vi "Client.vi"() -> ()   [LabVIEW 2021]
doc: "This VI acts as a client for an incoming websockets connection. Receives/sends string data to the connected client."
uses:
  StatusCode.ctl
  LV WebSockets.lvlib
panel:
  out "Status Code":T1=1000 items=["Normal Closure"=1000, "Going Away"=1001, "Protocol Error"=1002, "Wrong Data Type"=1003, "Reserved 1004"=1004, "Reserved 1005"=1005, "Reserved 1006"=1006, "Non Consistent Data Type"=1007, "Policy Violation"=1008, "Message Too Big"=1009, "Extensions Negotiation Error"=1010, "Unexpected Condition"=1011, "Reserved 1015"=1015]
  out "Close Reason":string
  in  "WS URI":string="ws://localhost:6123/resource/name"
  out "Resource Name":string
  out "HTTP Headers":variant
  in  "Stop":bool
  out "Received Data":string
  in  "Send":bool
  in  "Data":string
  # "WebSockets Example Client"
  # "This VI is a simple example of sending/receiving data using WebSockets.\nIt opens a WebSockets connection on Port 6123 and\nthen displays incoming string data. Strings can also be sent back to the client.\n\nInstructions for use:\n1) Run the SingleConnection.vi VI\n2) Set a suitable websocket URI including a resource name matching the one defined on the server\n2) Quickly run this VI"
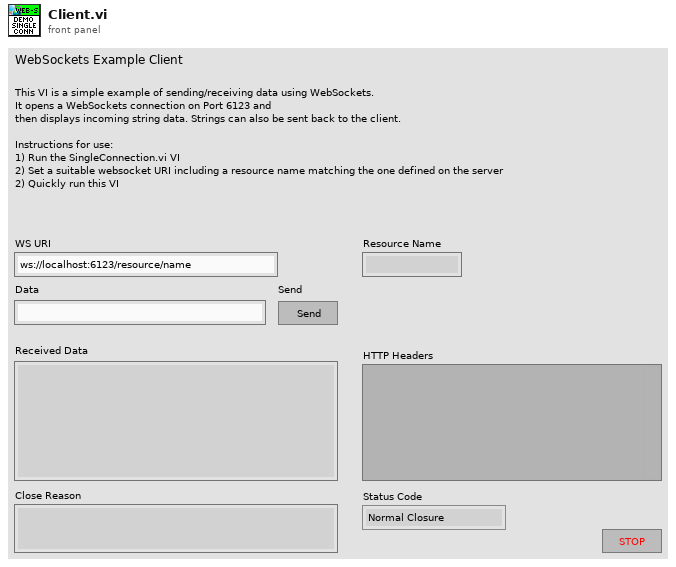
[diagram p1: front panel]
types:
  T1 = typedef "LV WebSockets.lvlib/StatusCode.ctl" = u16
  T2 = typedef "LV WebSockets.lvlib/Opcode.ctl" = enum8{"Continuation Frame", "Text Frame", "Binary Frame", "Reserved 3", "Reserved 4", "Reserved 5", "Reserved 6", "Reserved 7", "Connection Close", "Ping", "Pong", "Reserved B", "Reserved C", "Reserved D", "Reserved F"}
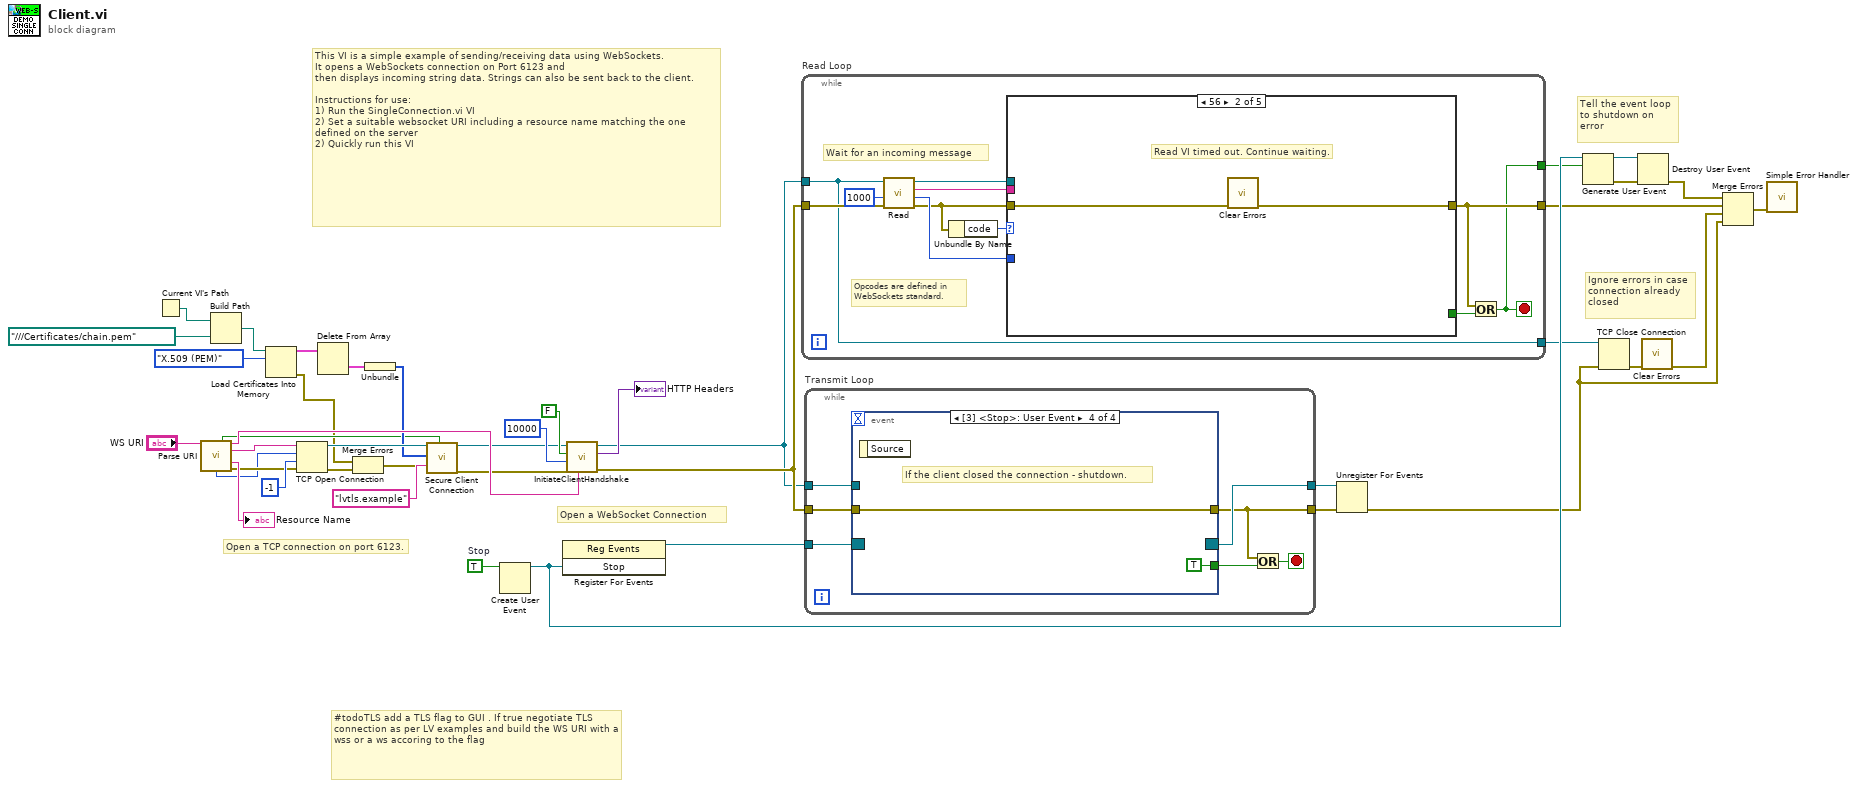
[diagram p0: block diagram]
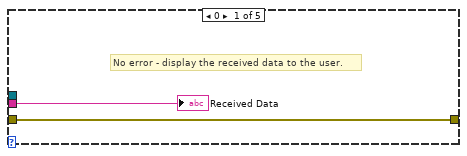
[diagram p2: hidden frame]
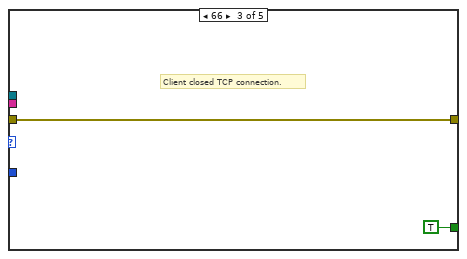
[diagram p3: hidden frame]
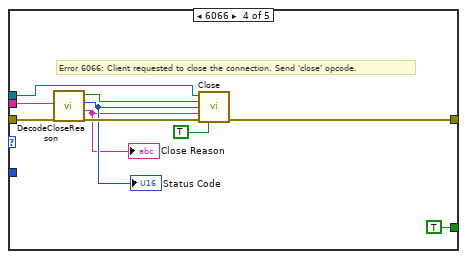
[diagram p4: hidden frame]
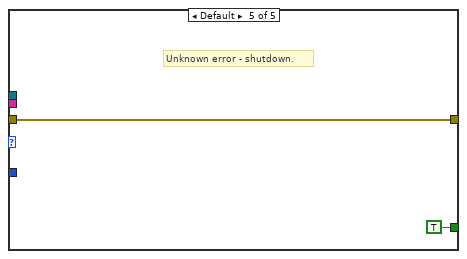
[diagram p5: hidden frame]
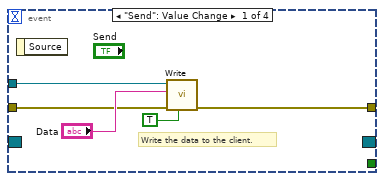
[diagram p6: hidden frame]
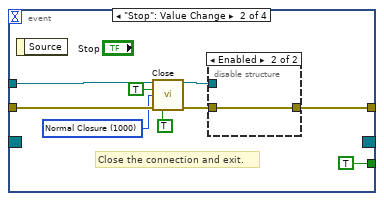
[diagram p7: hidden frame]
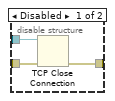
[diagram p8: hidden frame]
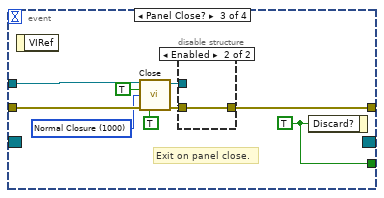
[diagram p9: hidden frame]
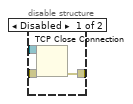
[diagram p10: hidden frame]
diagram:
  w40 = TRUE  # Stop
  # "#todoTLS add a TLS flag to GUI . If true negotiate TLS connection as per LV examples and build the WS URI with a wss or a ws accoring to the flag"
  # "Ignore errors in case\nconnection already\nclosed"
  # "Tell the event loop to shutdown on error"
  # "This VI is a simple example of sending/receiving data using WebSockets.\nIt opens a WebSockets connection on Port 6123 and\nthen displays incoming string data. Strings can also be sent back to the client.\n\nInstructions for use:\n1) Run the SingleConnection.vi VI\n2) Set a suitable websocket URI including a resource name matching the one defined on the server\n2) Quickly run this VI"
  # "Open a WebSocket Connection"
  # "Open a TCP connection on port 6123."
  n1 = Current VI's Path() -> (path=w3:path)
  n2 = call "Parse URI.vi"("URI"="WS URI") -> ("Secure"=w4:bool, "URI Out"=w24:string, "Hostname"=w23:string, "Resource Name"=→"Resource Name":string, "Port"=w19:u16, "error out"=w21:errorcluster)  [unwired: 7 in, 2 out]
  n3 = Build Path(base path=w3, name or relative path=path "../../../Certificates/chain.pem" ("cert chain")) -> (appended path=w13:path)
  n4 = Load Certificates Into Memory(10:enum32{"X.509 (PEM)"}."X.509 (PEM)" ("format"), 11:w13) -> (0:w1:errorcluster, 3:w6:cluster{"certificate":u8[]}[])  [unwired: 1 in]
  n5 = TCP Open Connection(address=w23, remote port or service name=w19, timeout ms (60000)=-1 ("timeout ms (25000)"), error in (no error)=w21) -> (connection ID=w9:refnum<k5>, error out=w12:errorcluster)  [unwired: 1 in]
  n6 = Delete From Array(array=w6) -> (deleted portion=w7:cluster{"certificate":u8[]})  [unwired: 2 in, 1 out]
  n7 = Merge Errors(w1, w12) -> (w2:errorcluster)
  n8 = Unbundle(w7) -> ("certificate"=w5:u8[])
  n9 = call "Secure Client Connection.vi"("TCP connection"=w9, "certificate"=w5, "server hostname"="lvtls.example" ("expected server hostname (must be \"lvtls.example\")"), "error in"=w2, "Secure the Connection (T)"=w4) -> ("TCP connection out"=w10:refnum<k5>, "error out"=w11:errorcluster)  [unwired: 12 in, 1 out]
  n10 = Create User Event(user event datatype=w40) -> (user event=w38:refnum<user-event>)  [unwired: 1 in, 1 out]
  n11 = register-events(w38) -> (reference out=w41:refnum<event-registration>)  [unwired: 2 in, 1 out]
  n12 = call "InitiateClientHandshake.vi"("WS URI"=w24, "error in (no error)"=w11, "timeout ms (5000)"=10000 ("timeout ms (25000)"), "Relative URI Request (F)"=FALSE, "WebSocket Connection in"=w10) -> ("error out"=w29:errorcluster, "Return Headers Out"=→"HTTP Headers":variant, "WebSocket Connection out"=w27:refnum<k5>)  [unwired: 4 in]
  n13 = while "Read Loop" {
    tunnel: w27 -> [w43]
    tunnel: [w44] -> w37
    tunnel: [w46] -> w28
    tunnel: w29 -> [w47]
    tunnel: [w43] -> w16
    stop <- w44 stop-if-true
    # "Wait for an incoming message"
    # "Opcodes are defined in\nWebSockets standard."
    n14 = call "Read.vi"("error in (no error)"=w47, "timeout ms (5000)"=1000 ("timeout ms (25000)"), "WebSocket Connection in"=w43) -> ("error out"=w48:errorcluster, "Opcode out"=w49:T2, "Data"=w51:string, "WebSocket Connection out"=w50:refnum<k5>)  [unwired: 5 in]
    n15 = Unbundle By Name(w48) -> ("code"=w52:i32)
    n16 = case shown="56" w52 {
      tunnel: w51 -> [w55 _ _ w64 _]
      tunnel: [_ _ TRUE TRUE TRUE] -> w45
      tunnel: w50 -> [_ _ _ w68 _]
      tunnel: w49 -> [_ _ _ _ _]
      tunnel: w48 -> [w54 w57 w58 w66 w69]
      tunnel: [w54 w56 w58 w65 w69] -> w46
      frame 0 {
        # "No error - display the received data to the user."
        "Received Data" <- w55
      }
      frame 56 {
        # "Read VI timed out. Continue waiting."
        n17 = call <vilib>:"Clear Errors.vi"("error in (no error)"=w57) -> ("error out"=w56:errorcluster)  [unwired: 5 in, 1 out]
      }
      frame 66 {
        # "Client closed TCP connection."
      }
      frame 6066 {
        # "Error 6066: Client requested to close the connection. Send 'close' opcode."
        n18 = call "DecodeCloseReason.vi"("Data"=w64) -> ("Reason"=w60:string, "Status Code"=w62:T1, "Close Reason Given"=w63:bool)  [unwired: 8 in]
        "Close Reason" <- w60
        "Status Code" <- w62
        n19 = call "Close.vi"("WebSocket Connection in"=w68, "Send Reason (F)"=w63, "Status Code"=w62, "Reason"=w60, "error in (no error)"=w66, "Mask payload?"=TRUE) -> ("error out"=w65:errorcluster)  [unwired: 8 in, 1 out]
      }
      frame Default {
        # "Unknown error - shutdown."
      }
    }
    n20 = Or(x=w46, y=w45) -> (x .or. y?=w44:bool)
  }
  n21 = while "Transmit Loop" {
    tunnel: w27 -> [w77]
    tunnel: w41 -> [w76]
    tunnel: [w75] -> w39
    tunnel: [w71] -> w30
    tunnel: w29 -> [w74]
    stop <- w72 stop-if-true
    n22 = event shown="[3] <Stop>: User Event" {
      selector: w76 -> [_ _ _ _]
      dyn-events: [_ _ _ _] -> w75
      timeout: _ -> [_ _ _ _]
      tunnel: w77 -> [w82 w90 w104 _]
      tunnel: [_ TRUE w102 TRUE] -> w73
      tunnel: [w79 w88 w100 w109] -> w71
      tunnel: w74 -> [w80 w86 w99 w109]
      event "Send": Value Change {
        # "Write the data to the client."
        n23 = event-data() -> ()  [unwired: 1 in, 1 out]
        n24 = call "Write.vi"("Mask payload?"=TRUE, "error in (no error)"=w80, "Data"="Data", "WebSocket Connection in"=w82) -> ("error out"=w79:errorcluster)  [unwired: 6 in, 1 out]
      }
      event "Stop": Value Change {
        w84 = T1 1000 items=["Normal Closure"=1000, "Going Away"=1001, "Protocol Error"=1002, "Wrong Data Type"=1003, "Reserved 1004"=1004, "Reserved 1005"=1005, "Reserved 1006"=1006, "Non Consistent Data Type"=1007, "Policy Violation"=1008, "Message Too Big"=1009, "Extensions Negotiation Error"=1010, "Unexpected Condition"=1011, "Reserved 1015"=1015] ("Status Code")
        # "Close the connection and exit."
        n25 = event-data() -> ()  [unwired: 1 in, 1 out]
        n26 = call "Close.vi"("WebSocket Connection in"=w90, "Send Reason (F)"=TRUE, "Status Code"=w84, "error in (no error)"=w86, "Mask payload?"=TRUE) -> ("WebSocket Connection in"=w89:refnum<k5>, "error out"=w87:errorcluster)  [unwired: 9 in]
        n27 = disable-structure shown="Enabled" {
          disable-tunnel: w89 -> [w94 _]
          disable-tunnel: [w93 w95] -> w88
          disable-tunnel: w87 -> [w92 w95]
          frame Disabled {
            n28 = TCP Close Connection(connection ID=w94, error in (no error)=w92) -> (error out=w93:errorcluster)  [unwired: 1 in, 1 out]
          }
          frame Enabled {
          }
        }
      }
      event Panel Close? {
        w97 = T1 1000 items=["Normal Closure"=1000, "Going Away"=1001, "Protocol Error"=1002, "Wrong Data Type"=1003, "Reserved 1004"=1004, "Reserved 1005"=1005, "Reserved 1006"=1006, "Non Consistent Data Type"=1007, "Policy Violation"=1008, "Message Too Big"=1009, "Extensions Negotiation Error"=1010, "Unexpected Condition"=1011, "Reserved 1015"=1015] ("Status Code")
        w102 = TRUE ("Discard?")
        # "Exit on panel close."
        n29 = event-data() -> ()  [unwired: 1 in, 1 out]
        n30 = call "Close.vi"("WebSocket Connection in"=w104, "Send Reason (F)"=TRUE, "Status Code"=w97, "error in (no error)"=w99, "Mask payload?"=TRUE) -> ("WebSocket Connection in"=w103:refnum<k5>, "error out"=w101:errorcluster)  [unwired: 9 in]
        n31 = disable-structure shown="Enabled" {
          disable-tunnel: w103 -> [w107 _]
          disable-tunnel: w101 -> [w106 w108]
          disable-tunnel: [w105 w108] -> w100
          frame Disabled {
            n32 = TCP Close Connection(connection ID=w107, error in (no error)=w106) -> (error out=w105:errorcluster)  [unwired: 1 in, 1 out]
          }
          frame Enabled {
          }
        }
        n33 = event-data("Discard?"=w102) -> ()  [unwired: 1 in, 1 out]
      }
      event User Event {
        # "If the client closed the connection - shutdown."
        n34 = event-data() -> ()  [unwired: 1 in, 1 out]
      }
    }
    n35 = Or(x=w71, y=w73) -> (x .or. y?=w72:bool)
  }
  n36 = Unregister For Events(event registration refnum=w39, error in=w30) -> (error out=w17:errorcluster)
  n37 = Generate User Event(user event=w38, event data cluster=w37) -> (user event out=w36:refnum<user-event>, error out=w35:errorcluster)  [unwired: 2 in]
  n38 = TCP Close Connection(connection ID=w16, error in (no error)=w17) -> (error out=w26:errorcluster)  [unwired: 1 in, 1 out]
  n39 = Destroy User Event(user event=w36, error in=w35) -> (error out=w34:errorcluster)
  n40 = call <vilib>:"Clear Errors.vi"("error in (no error)"=w26) -> ("error out"=w18:errorcluster)  [unwired: 5 in, 1 out]
  n41 = Merge Errors(w34, w28, w18, w17) -> (w31:errorcluster)
  n42 = call <vilib>:"Simple Error Handler.vi"("error in (no error)"=w31) -> ()  [unwired: 4 in, 5 out]
